vi "RemoveHardware.vi"(8 "error in (no error)":errorcluster, 11 "Microscope in":refnum<class "Microscope.lvclass">) -> (0 "error out":errorcluster, 3 "Microscope out":refnum<class "Microscope.lvclass">)   [LabVIEW 2020, in "Microscope.lvlib" / "Microscope.lvclass"]
uses:
  Microscope.lvclass
  Microscope.lvclass/Microscope.ctl
  <vilib>/ActorFramework/Message Enqueuer/Message Enqueuer.lvclass/Message Enqueuer.ctl
  <vilib>/ActorFramework/Message Enqueuer/Enqueue.vi
  <vilib>/ActorFramework/Stop Msg/Stop Msg.lvclass
  C:/Program Files/National Instruments/LabVIEW 2020/vi.lib/ActorFramework/Message/Message.lvclass
  <vilib>/ActorFramework/Message Priority Queue/Priority Enqueue.vi
panel:
  out "key not found?":bool
  in  "Label":string
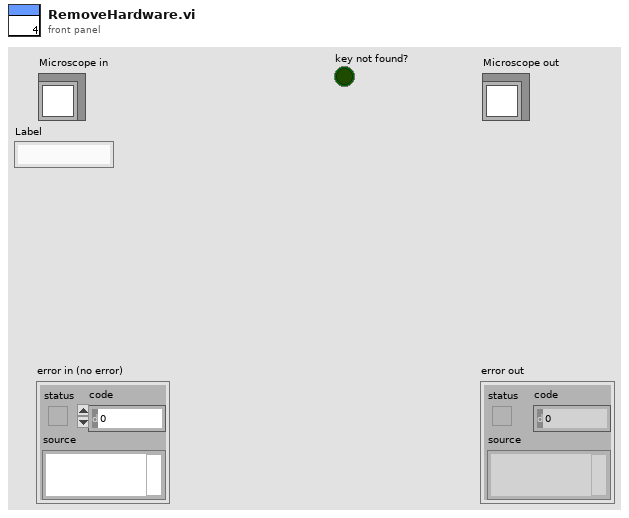
[diagram p1: front panel]
types:
  T1 = map{string, refnum<class "GenericController.lvclass">}
  T2 = map{string, refnum<class "Message Enqueuer.lvclass">}
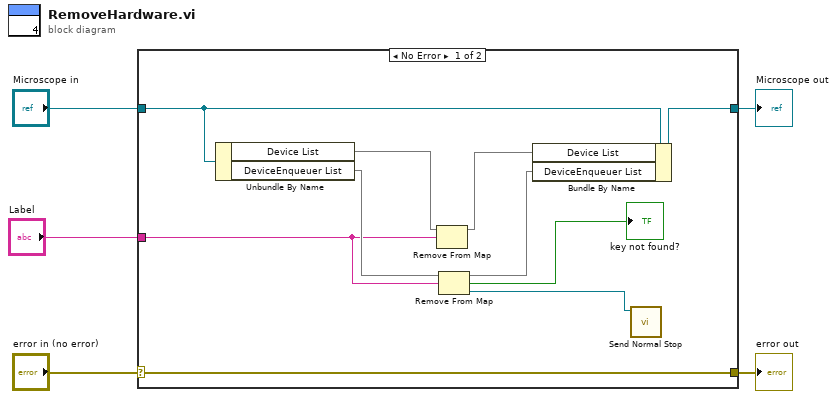
[diagram p0: block diagram]
diagram:
  n1 = case shown="No Error" "error in (no error)" {
    selector: "error in (no error)" -> [w15 w17]
    tunnel: [w15 w17] -> w4
    tunnel: [w13 w16] -> w2
    tunnel: "Microscope in" -> [w14 w16]
    tunnel: "Label" -> [w8 _]
    frame No Error {
      n2 = Unbundle By Name(w14) -> ("Device List"=w12:T1, "DeviceEnqueuer List"=w10:T2)
      n3 = Remove From Map(10:w8, 11:w12) -> (3:w11:T1)  [unwired: 2 out]
      n4 = Remove From Map(10:w8, 11:w10) -> (1:w6:refnum<class "Message Enqueuer.lvclass">, 2:→"key not found?":bool, 3:w9:T2)
      n5 = Bundle By Name(cluster=w14, "Device List"=w11, "DeviceEnqueuer List"=w9) -> (w13:refnum<class "Microscope.lvclass">)
      n6 = call <vilib>:"Send Normal Stop.vi"("Message Enqueuer"=w6) -> ()  [unwired: 10 in, 1 out]
    }
    frame Error {
    }
  }
  "error out" <- w4
  "Microscope out" <- w2
